vi "Engine - GDI - Boost Actuation Host.vi"() -> ()   [LabVIEW 2015, in "ECS-Host.lvlib"]
uses:
  ECS-Host.lvlib
  <vilib>/addons/Software Calibration Management/XControls/TBL1D.xctl
panel:
  out "WgPsnStp":sgl caption="[%Open]"
  out "WgDutyCyc_TblOut":sgl caption="[%]"
  out "WgDutyCyc_Des":sgl caption="[%]"
  in  "WgDutyCyc_Tbl":cluster{"X":sgl[], "Y":sgl[]}(xcontrol)
  in  "WgPWM_E":bool
  in  "WgPWMFreq":sgl caption="[Hz]"
  in  "WgDutyCyc_ManE":bool
  in  "WgDutyCyc_Man":sgl caption="[%]"
  in  "WgDutyCyc_Min":sgl caption="[%]"
  in  "WgDutyCyc_Max":sgl caption="[%]"
  out "BPVPsnStp":sgl caption="[%Open]"
  out "BPVDutyCyc_TblOut":sgl caption="[%]"
  out "BPVDutyCyc_Des":sgl caption="[%]"
  in  "BPVDutyCyc_Tbl":cluster{"X":sgl[], "Y":sgl[]}(xcontrol)
  in  "BPVPWM_E":bool
  in  "BPVPWMFreq":sgl caption="[Hz]"
  in  "BPVDutyCyc_ManE":bool
  in  "BPVDutyCyc_Man":sgl caption="[%]"
  in  "BPVDutyCyc_Min":sgl caption="[%]"
  in  "BPVDutyCyc_Max":sgl caption="[%]"
  # "Turbo Bypass Valve (BPV) Actuator"
  # "Wastegate (Wg) Actuator"
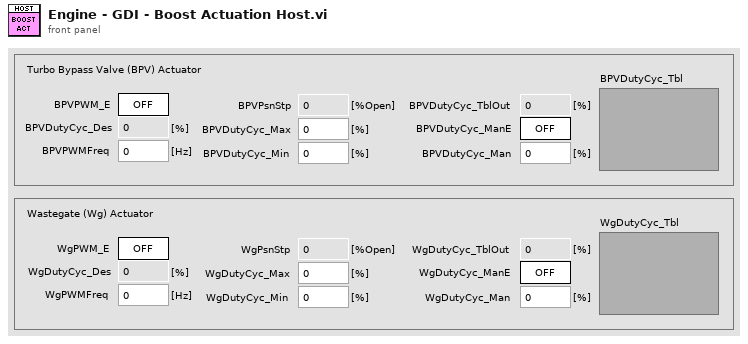
[diagram p1: front panel]
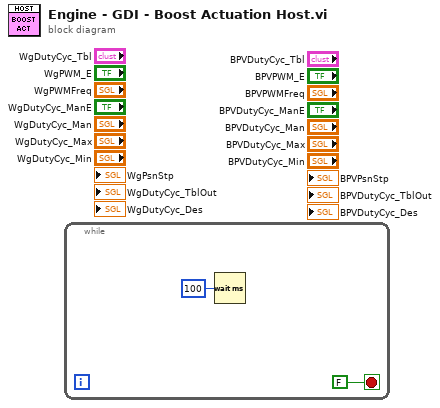
[diagram p0: block diagram]
diagram:
  n1 = while {
    stop <- FALSE stop-if-true
    n2 = Wait (ms)(milliseconds to wait=u32 100) -> ()  [unwired: 1 out]
  }
